vi "Run.vi"(8 "error in (no error)":errorcluster, 11 "LUnit Inheriting Test Case In":refnum<class "LUnit Inheriting Test Case.lvclass">) -> (0 "error out":errorcluster, 1 "Done?":bool, 2 "Results":T1(array[cluster]), 3 "LUnit Inheriting Test Case Out":refnum<class "LUnit Inheriting Test Case.lvclass">)   [LabVIEW 2020, in "LUnit Inheriting Test Case.lvclass"]
doc: "Execute test and return result."
uses:
  LUnit Inheriting Test Case.lvclass
  <vilib>/Astemes/LUnit/Test Case.lvclass
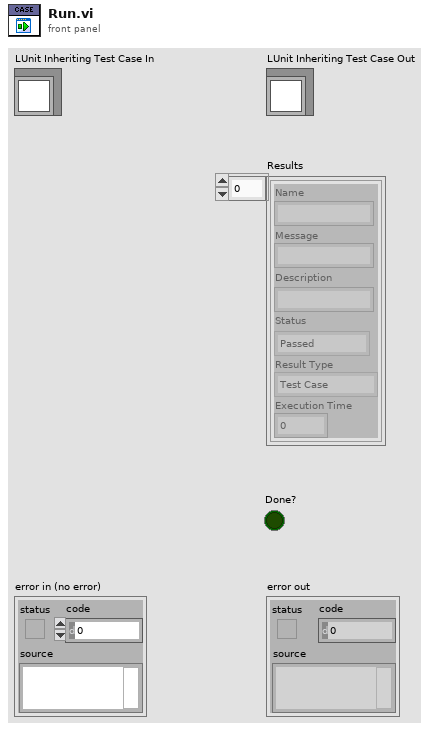
[diagram p1: front panel]
types:
  T1 = cluster{"Name":string, "Message":string, "Description":string, "Status":enum16{"", "Passed", "Failed", "Error", "Skipped", "Setup Error", "Broken", "Teardown Error"}, "Result Type":enum16{"Test Case", "Test Suite", "Test Run", "Pass", "Fail", "Skip", "Pass if", "Fail if", "Pass if Error", "Fail if Error", "Pass if Equal", "Fail if Equal"}, "Execution Time":dbl}[]
  T2 = typedef "Semaphore RefNum" = refnum<k1>
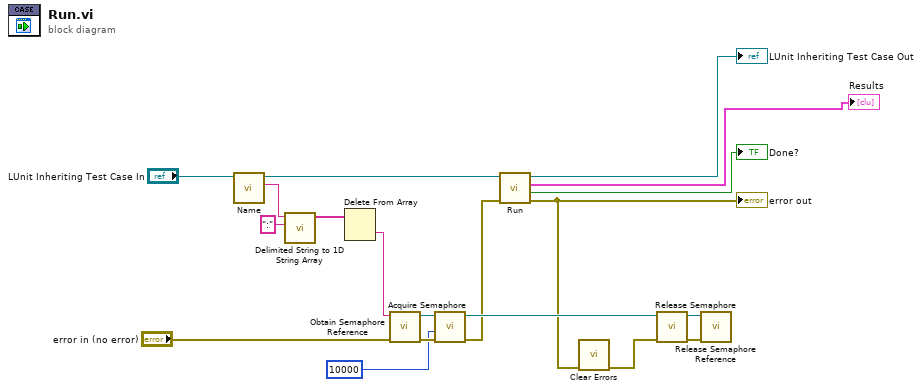
[diagram p0: block diagram]
diagram:
  n1 = call-dynamic "Name.vi"("LUnit Test Case in"="LUnit Inheriting Test Case In") -> ("Name"=w5:string, "LUnit Test Case out"=w6:refnum<class "LUnit Inheriting Test Case.lvclass">)  [unwired: 8 in, 1 out]
  n2 = call <vilib>:"Delimited String to 1D String Array.vi"("delimiter"=":", "delimited string"=w5) -> ("string array"=w3:string[])  [unwired: 9 in]
  n3 = Delete From Array(array=w3) -> (deleted portion=w2:string)  [unwired: 2 in, 1 out]
  n4 = call <vilib>:"Obtain Semaphore Reference.vi"("error in (no error)"="error in (no error)", "name (unnamed)"=w2) -> ("error out"=w16:errorcluster, "semaphore"=w17:T2)  [unwired: 3 in, 1 out]
  n5 = call <vilib>:"Acquire Semaphore.vi"("error in (no error)"=w16, "ms timeout (-1)"=10000, "semaphore"=w17) -> ("error out"=w10:errorcluster, "semaphore out"=w15:T2)  [unwired: 2 in, 1 out]
  n6 = call-parent "Run.vi"("error in (no error)"=w10, "LUnit Test Case In"=w6) -> ("error out"=w8:errorcluster, "Done?"=→"Done?":bool, "Results"=→"Results":T1, "LUnit Test Case Out"=→"LUnit Inheriting Test Case Out":refnum<class "LUnit Inheriting Test Case.lvclass">)  [unwired: 6 in]
  "error out" <- w8
  n7 = call <vilib>:"Clear Errors.vi"("error in (no error)"=w8) -> ("error out"=w12:errorcluster)  [unwired: 5 in, 1 out]
  n8 = call <vilib>:"Release Semaphore.vi"("error in (no error)"=w12, "semaphore"=w15) -> ("error out"=w13:errorcluster, "semaphore out"=w14:T2)  [unwired: 4 in]
  n9 = call <vilib>:"Release Semaphore Reference.vi"("error in (no error)"=w13, "semaphore"=w14) -> ()  [unwired: 8 in, 2 out]
